vi "GOMDBTS2048 calibration sample.vi"() -> ()   [LabVIEW 2009]
panel:
  out "function return 8":i32
  out "function return 7":i32
  out "function return 6":i32
  out "function return 5":i32
  out "function return 4":i32
  out "function return 3":i32
  out "function return 2":i32
  out "function return":i32
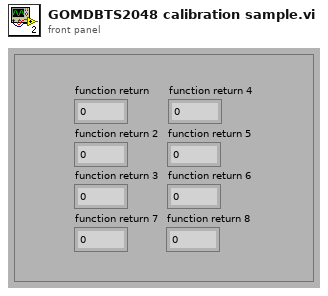
[diagram p1: front panel]
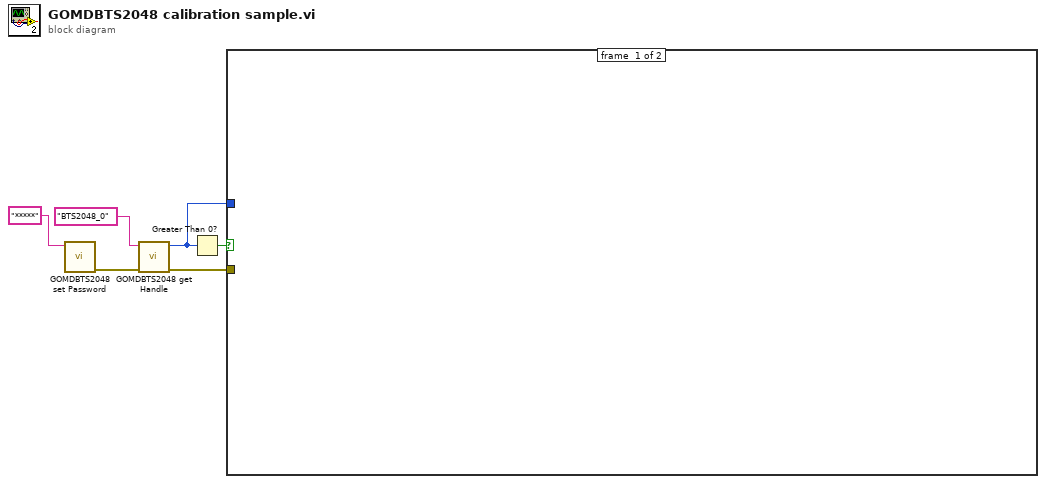
[diagram p0: block diagram]
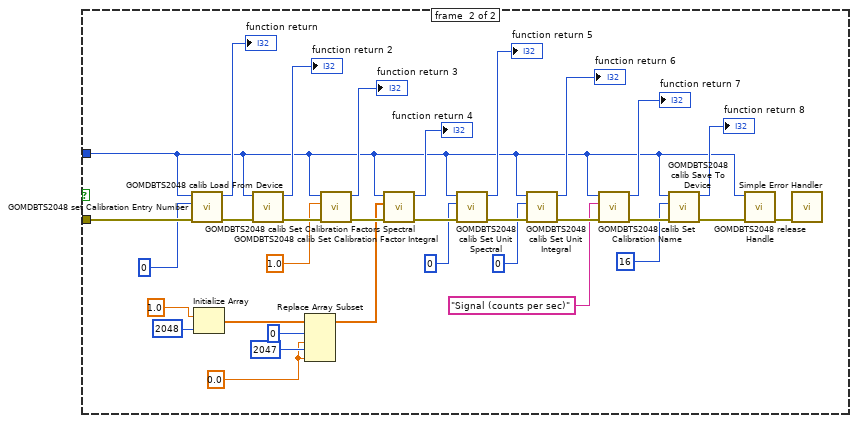
[diagram p2: hidden frame]
diagram:
  n1 = call <userlib>:"GOMDBTS2048 set Password.vi"("value"="*****" ("deviceName")) -> ("error out"=w5:errorcluster)  [unwired: 9 in, 1 out]
  n2 = call <userlib>:"GOMDBTS2048 get Handle.vi"("error in (no error)"=w5, "device"="BTS2048_0" ("deviceName")) -> ("error out"=w4:errorcluster, "handle"=w1:i32)  [unwired: 7 in, 1 out]
  n3 = Greater Than 0?(x=w1) -> (x > 0?=w6:bool)
  n4 = case shown="True" w6 {
    tunnel: w4 -> [_ w38]
    tunnel: w1 -> [_ w13]
    frame #0 {
    }
    frame #1 {
      w8 = 0.0 ("element")
      n5 = call <userlib>:"GOMDBTS2048 set Calibration Entry Number.vi"("error in (no error)"=w38, "calibrationEntryNumber"=0, "handle"=w13) -> ("error out"=w36:errorcluster, "function return"=→"function return":i32)  [unwired: 7 in]
      n6 = Initialize Array(1.0 ("element"), 2048 ("dimension size")) -> (w11:dbl[])
      n7 = call <userlib>:"GOMDBTS2048 calib Load From Device.vi"("error in (no error)"=w36, "handle"=w13) -> ("error out"=w35:errorcluster, "function return"=→"function return 2":i32)  [unwired: 8 in]
      n8 = Replace Array Subset(array=w11, new element #1=w8, index #1=0 ("index"), new element #2=w8, index #2=2047 ("index")) -> (w7:dbl[])
      n9 = call <userlib>:"GOMDBTS2048 calib Set Calibration Factor Integral.vi"("error in (no error)"=w35, "value"=1.0, "handle"=w13) -> ("error out"=w24:errorcluster, "function return"=→"function return 3":i32)  [unwired: 7 in]
      n10 = call <userlib>:"GOMDBTS2048 calib Set Calibration Factors Spectral.vi"("error in (no error)"=w24, "values"=w7, "handle"=w13) -> ("error out"=w22:errorcluster, "function return"=→"function return 4":i32)  [unwired: 7 in]
      n11 = call <userlib>:"GOMDBTS2048 calib Set Unit Spectral.vi"("error in (no error)"=w22, "value"=0, "handle"=w13) -> ("error out"=w23:errorcluster, "function return"=→"function return 5":i32)  [unwired: 7 in]
      n12 = call <userlib>:"GOMDBTS2048 calib Set Unit Integral.vi"("error in (no error)"=w23, "value"=0, "handle"=w13) -> ("error out"=w34:errorcluster, "function return"=→"function return 6":i32)  [unwired: 7 in]
      n13 = call <userlib>:"GOMDBTS2048 calib Set Calibration Name.vi"("error in (no error)"=w34, "value"="Signal (counts per sec)", "handle"=w13) -> ("error out"=w33:errorcluster, "function return"=→"function return 7":i32)  [unwired: 7 in]
      n14 = call <userlib>:"GOMDBTS2048 calib Save To Device.vi"("error in (no error)"=w33, "configNumber"=16, "handle"=w13) -> ("error out"=w14:errorcluster, "function return"=→"function return 8":i32)  [unwired: 7 in]
      n15 = call <userlib>:"GOMDBTS2048 release Handle.vi"("error in (no error)"=w14, "handle"=w13) -> ("error out"=w12:errorcluster)  [unwired: 8 in, 1 out]
      n16 = call <vilib>:"Simple Error Handler.vi"("error in (no error)"=w12) -> ()  [unwired: 4 in, 5 out]
    }
  }
